vi "Seq Dialog Check Goto using RSLinx Tag Boolean.vi"(8 "Segment Data":T3) -> (0 "Step Hisitory":string[](array[string]), 2 "Segment Data 2":T3)   [LabVIEW 2018]
uses:
  type defs/plc path and tag.ctl
  <vilib>/Platform/dataskt.llb/DataSocket Reference Type.ctl
  type defs/Sequence Info.ctl
  type defs/sequence goto step params.ctl
panel:
  in  "goto step":u8=159
  in  "goto if...":bool
  in  "Tag String":T1={"Tag Name"="S060.PXI.Signals.PlltData.SN", "Network Path"="172.15.51.1,1,0", "use opc"=FALSE, "DataSocket Reference"={"CWDSLib._DCWDataSocket"=refnum, "CWDSLib._DCWData"=refnum, "OnDataUpdated"=0, "OnStatusUpdated"=0}} {"DataSocket Reference"."OnStatusUpdated" format="%.0x"; "DataSocket Reference"."OnDataUpdated" format="%.0x"}
  out "Name":string="Pre Run Station - Glass - Vent Open"
  in  "Description":string
  in  "Save":bool
  in  "Cancel":bool
  # "Goto step"
  # "if"
  # "="
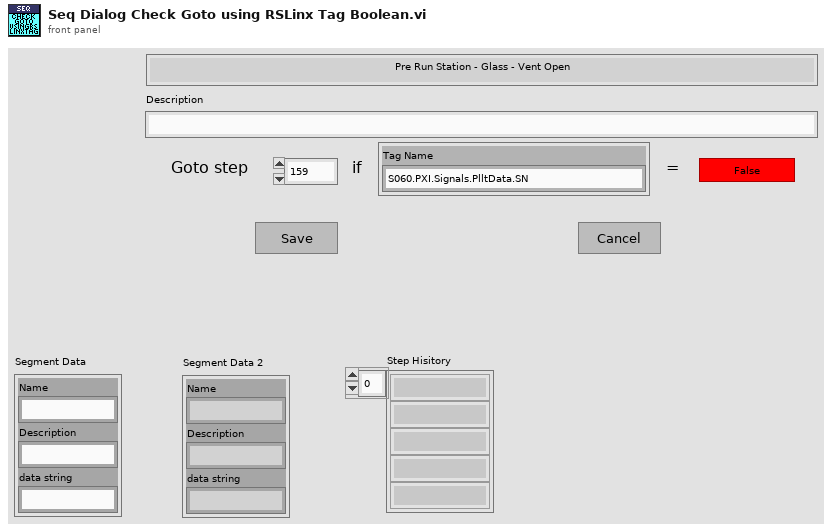
[diagram p1: front panel]
types:
  T1 = typedef "plc path and tag.ctl" = cluster{"Tag Name":string, "Network Path":string, "use opc":bool, "DataSocket Reference":T2}
  T2 = typedef "DataSocket Reference Type.ctl" = cluster{"CWDSLib._DCWDataSocket":refnum<k7>, "CWDSLib._DCWData":refnum<k7>, "OnDataUpdated":u32, "OnStatusUpdated":u32}
  T3 = typedef "Sequence Info.ctl" = cluster{"Name":string, "Description":string, "data string":string}
  T4 = typedef "sequence goto step params.ctl" = cluster{"Data Boolean":bool, "PLC Path and Tag":T1, "goto step":u8}
  T5 = cluster{"Segment Data":T3, "Old Data":string, "New Data":string, "sequence goto step params":T4}
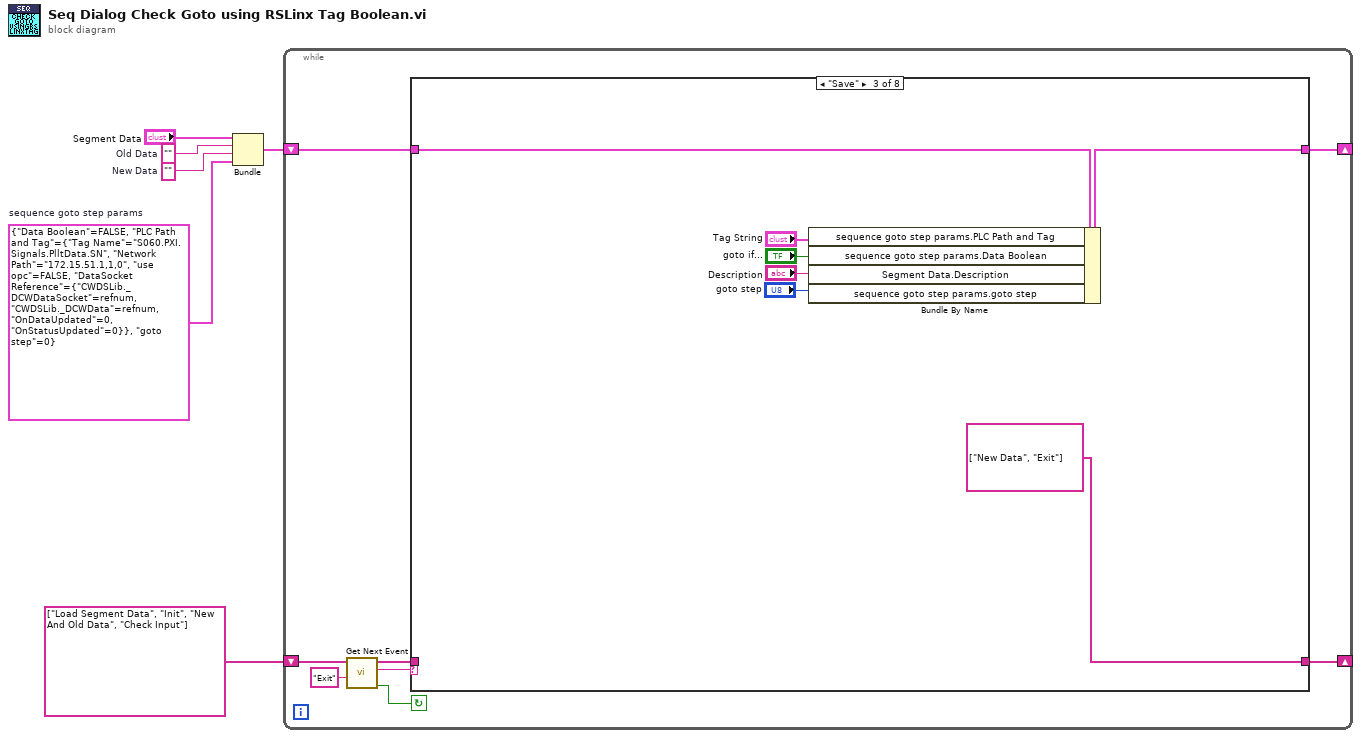
[diagram p0: block diagram]
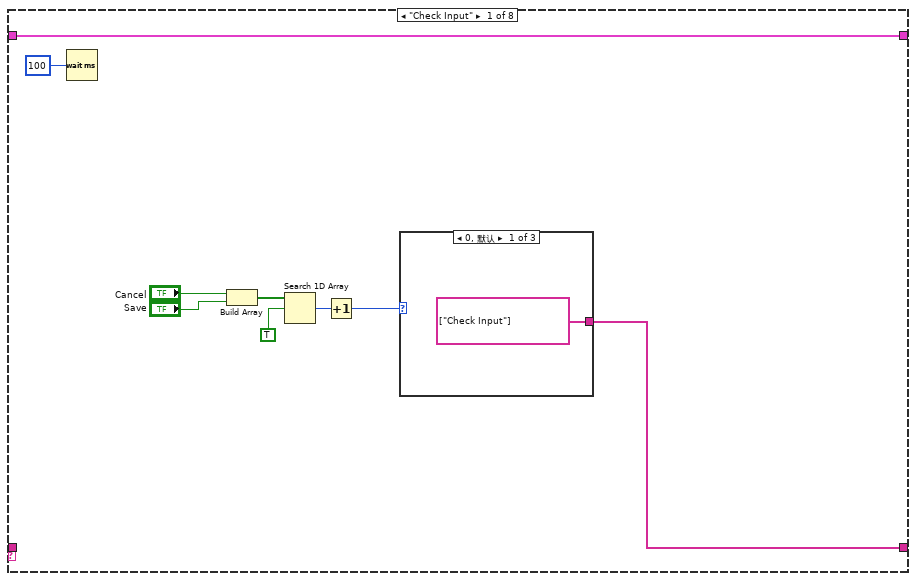
[diagram p2: hidden frame]
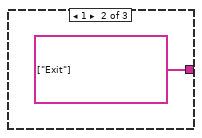
[diagram p3: hidden frame]
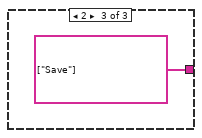
[diagram p4: hidden frame]
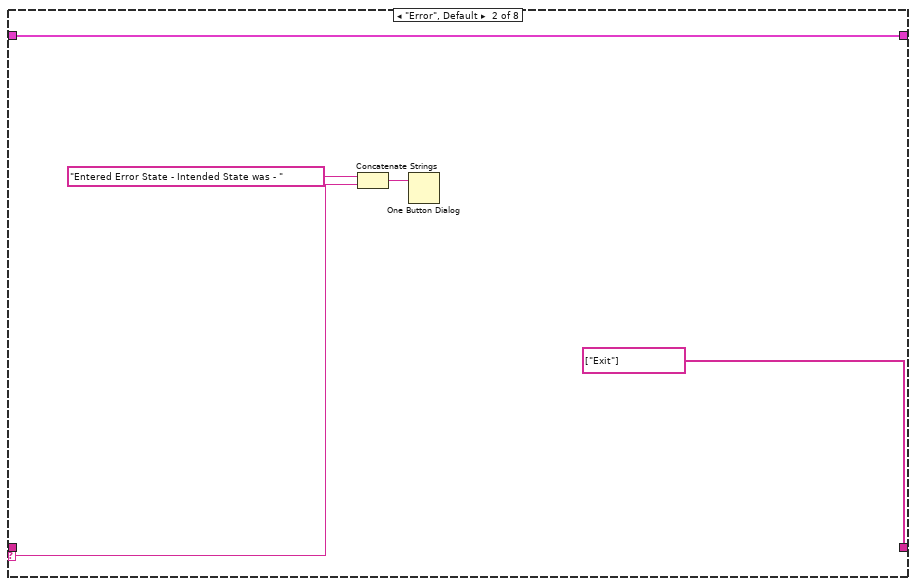
[diagram p5: hidden frame]
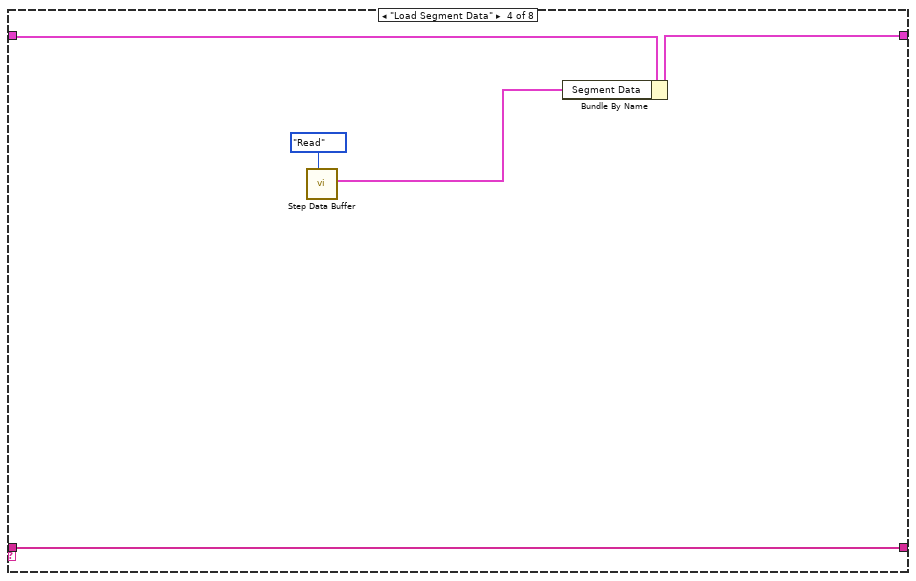
[diagram p6: hidden frame]
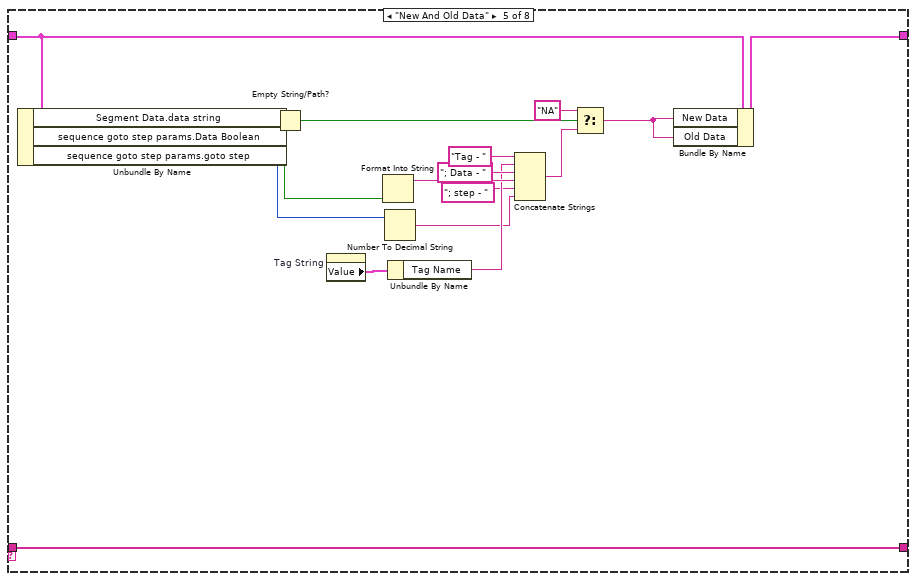
[diagram p7: hidden frame]
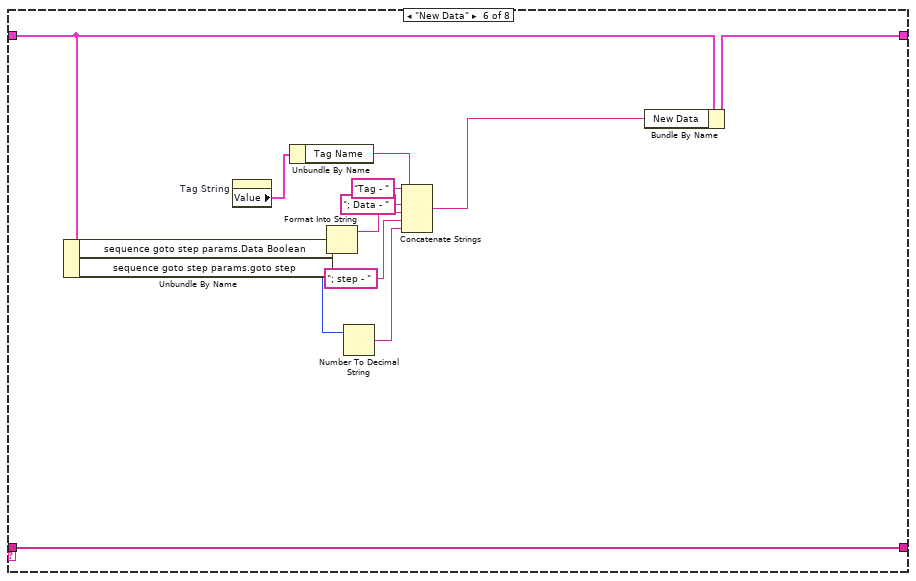
[diagram p8: hidden frame]
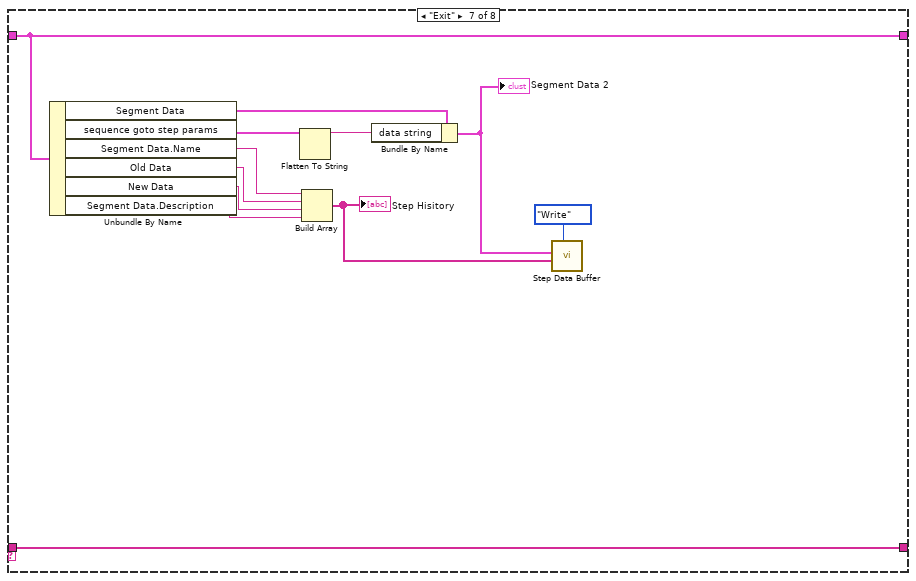
[diagram p9: hidden frame]
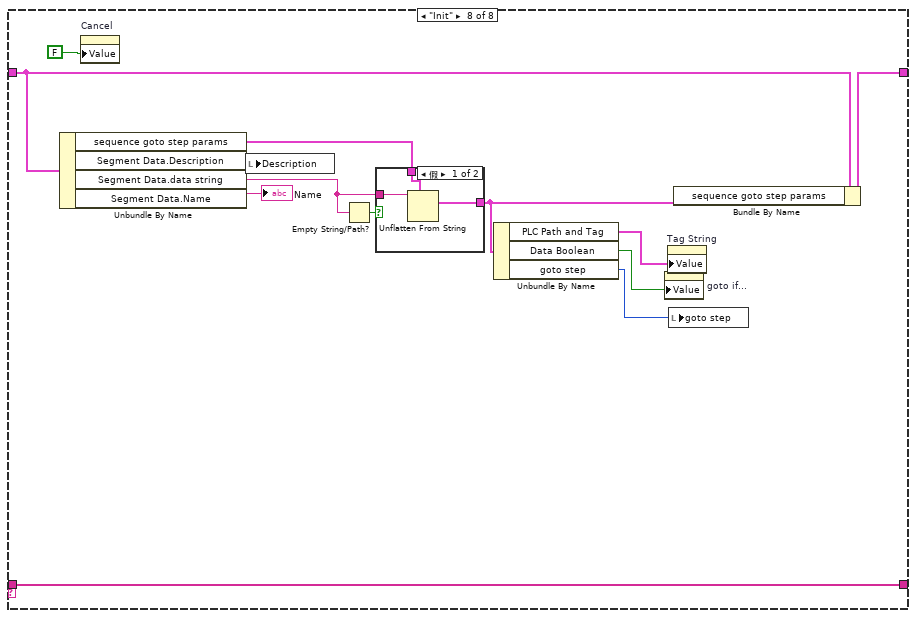
[diagram p10: hidden frame]
diagram:
  w1 = T4 {"Data Boolean"=FALSE, "PLC Path and Tag"={"Tag Name"="S060.PXI.Signals.PlltData.SN", "Network Path"="172.15.51.1,1,0", "use opc"=FALSE, "DataSocket Reference"={"CWDSLib._DCWDataSocket"=refnum, "CWDSLib._DCWData"=refnum, "OnDataUpdated"=0, "OnStatusUpdated"=0}}, "goto step"=0}  # sequence goto step params
  w3 = ""  # New Data
  w4 = ""  # Old Data
  n1 = Bundle("Segment Data"="Segment Data", "Old Data"=w4, "New Data"=w3, "sequence goto step params"=w1) -> (w6:T5)  [unwired: 1 in]
  n2 = while {
    shift-right: [w12] -> _
    shift-left: string[] ["Load Segment Data", "Init", "New And Old Data", "Check Input"] ("Event queue out") -> [w11]
    shift-right: [w7] -> _
    shift-left: w6 -> [w8]
    stop <- w10 continue-if-true
    n3 = call "Get Next Event.vi"("Exit Event"="Exit", "event queue in"=w11) -> ("Condition (Exit:F)"=w10:bool, "next event"=w14:string, "event queue out"=w13:string[])  [unwired: 3 in]
    n4 = case shown="\"Save\"" w14 {
      selector: w14 -> [_ w29 _ _ _ _ _ _]
      tunnel: w13 -> [_ _ _ w39 w54 w73 w85 w98]
      tunnel: [w17 string[] ["Exit"] ("event queue out") string[] ["New Data", "Exit"] ("Event queue out") w39 w54 w73 w85 w98] -> w12
      tunnel: w8 -> [w22 w27 w37 w41 w56 w72 w84 w94]
      tunnel: [w22 w27 w38 w40 w55 w71 w84 w91] -> w7
      frame "Check Input" {
        n5 = Wait (ms)(milliseconds to wait=u32 100) -> ()  [unwired: 1 out]
        n6 = Build Array("Cancel", "Save") -> (w19:bool[])
        n7 = Search 1D Array(1D array=w19, element=TRUE) -> (index of element=w20:i32)  [unwired: 1 in]
        n8 = Increment(x=w20) -> (x+1=w21:i32)
        n9 = case shown="0, 默认" w21 {
          tunnel: [string[] ["Check Input"] ("Events to Insert") string[] ["Exit"] ("Events to Insert") string[] ["Save"] ("Events to Insert")] -> w17
          frame 0, Default {
          }
          frame 1 {
          }
          frame 2 {
          }
        }
      }
      frame "Error", Default {
        n10 = Concatenate Strings("Entered Error State - Intended State was - " ("string"), w29) -> (w31:string)
        n11 = One Button Dialog(message=w31) -> ()  [unwired: 1 in, 1 out]
      }
      frame "Save" {
        n12 = Bundle By Name(cluster=w37, "sequence goto step params.PLC Path and Tag"="Tag String", "sequence goto step params.Data Boolean"="goto if...", "Segment Data.Description"="Description", "sequence goto step params.goto step"="goto step") -> (w38:T5)
      }
      frame "Load Segment Data" {
        n13 = call "Step Data Buffer.vi"("Mode"=enum16{"Init", "Read", "Write"}."Read") -> ("Segment Data Out"=w43:T3)  [unwired: 6 in, 4 out]
        n14 = Bundle By Name(cluster=w41, "Segment Data"=w43) -> (w40:T5)
      }
      frame "New And Old Data" {
        n15 = Unbundle By Name(w56) -> ("Segment Data.data string"=w60:string, "sequence goto step params.Data Boolean"=w50:bool, "sequence goto step params.goto step"=w45:u8)
        n16 = Empty String/Path?(string/path=w60) -> (empty?=w57:bool)
        n17 = property on="Tag String" class="Clust (严格)"() -> ("Value"=w48:T1)  [unwired: 2 in, 2 out]
        n18 = Format Into String(w50) -> (resulting string=w49:string)  [unwired: 3 in, 1 out]
        n19 = Number To Decimal String(number=w45) -> (decimal integer string=w44:string)  [unwired: 1 in]
        n20 = Unbundle By Name(w48) -> ("Tag Name"=w47:string)
        n21 = Concatenate Strings("Tag - " ("string"), w47, "; Data - " ("string"), w49, "; step - " ("string"), w44) -> (w51:string)
        n22 = Select(t="NA", s=w57, f=w51) -> (s? t:f=w59:string)
        n23 = Bundle By Name(cluster=w56, "New Data"=w59, "Old Data"=w59) -> (w55:T5)
      }
      frame "New Data" {
        n24 = Unbundle By Name(w72) -> ("sequence goto step params.Data Boolean"=w67:bool, "sequence goto step params.goto step"=w63:u8)
        n25 = property on="Tag String" class="Clust (严格)"() -> ("Value"=w65:T1)  [unwired: 2 in, 2 out]
        n26 = Unbundle By Name(w65) -> ("Tag Name"=w64:string)
        n27 = Format Into String(w67) -> (resulting string=w66:string)  [unwired: 3 in, 1 out]
        n28 = Number To Decimal String(number=w63) -> (decimal integer string=w62:string)  [unwired: 1 in]
        n29 = Concatenate Strings("Tag - " ("string"), w64, "; Data - " ("string"), w66, "; step - " ("string"), w62) -> (w68:string)
        n30 = Bundle By Name(cluster=w72, "New Data"=w68) -> (w71:T5)
      }
      frame "Exit" {
        n31 = Unbundle By Name(w84) -> ("Segment Data"=w77:T3, "sequence goto step params"=w75:T4, "Segment Data.Name"=w83:string, "Old Data"=w82:string, "New Data"=w81:string, "Segment Data.Description"=w78:string)
        n32 = Flatten To String(anything=w75) -> (data string=w74:string)  [unwired: 3 in, 2 out]
        n33 = Build Array(w83, w82, w81, w78) -> (w79:string[])
        "Step Hisitory" <- w79
        n34 = Bundle By Name(cluster=w77, "data string"=w74) -> (w76:T3)
        "Segment Data 2" <- w76
        n35 = call "Step Data Buffer.vi"("Mode"=enum16{"Init", "Read", "Write"}."Write", "Step Hisitory In"=w79, "Segment Data In"=w76) -> ()  [unwired: 4 in, 5 out]
      }
      frame "Init" {
        n36 = Unbundle By Name(w94) -> ("sequence goto step params"=w88:T4, "Segment Data.Description"=w97:string, "Segment Data.data string"=w92:string, "Segment Data.Name"=→"Name":string)
        n37 = property on="Cancel" class="Bool (严格)"("Value"=FALSE ("Cancel")) -> ()  [unwired: 2 in, 2 out]
        n38 = local write "Description"(w97) -> ()
        n39 = Empty String/Path?(string/path=w92) -> (empty?=w93:bool)
        n40 = case shown="假" w93 {
          tunnel: w92 -> [w99 _]
          tunnel: w88 -> [w101 w102]
          tunnel: [w100 w102] -> w87
          frame False {
            n41 = Unflatten From String(type=w101, binary string=w99) -> (value=w100:T4)  [unwired: 3 in, 2 out]
          }
          frame True {
          }
        }
        n42 = Unbundle By Name(w87) -> ("PLC Path and Tag"=w90:T1, "Data Boolean"=w89:bool, "goto step"=w86:u8)
        n43 = property on="goto if..." class="Bool (严格)"("Value"=w89) -> ()  [unwired: 2 in, 2 out]
        n44 = property on="Tag String" class="Clust (严格)"("Value"=w90) -> ()  [unwired: 2 in, 2 out]
        n45 = local write "goto step"(w86) -> ()
        n46 = Bundle By Name(cluster=w94, "sequence goto step params"=w87) -> (w91:T5)
      }
    }
  }
